vi "fpga.vi"() -> ()   [LabVIEW 2016]
uses:
  <vilib>/rvi/Emulation/niFpgaGetClockAttributes.vi
  <vilib>/rvi/Emulation/niFpgaSctlEmulationGetInTimedLoop.vi
  <vilib>/rvi/Emulation/niFpgaEmulationReportErrorSimple.vi
  <vilib>/rvi/interface/RandomDataEmulation/niFpgaRandomDataHandleErrors.vi
  <vilib>/rvi/Emulation/niFpgaCriticalErrorInLSC.vi
  <vilib>/rvi/eio/common/nirviEmuTemplateMethod_errors.vi
  <vilib>/rvi/DataTransferAndStorage/Container/XNode/niFpgaContainer.xnode
  <vilib>/rvi/interface/RandomDataEmulation/nirviRandomDataFpgaReadWriteTemplate.vi
  <vilib>/eio/EIONode/EIONode.xnode
panel:
  out "bool_arr_out":bool[](array[boolean])
  in  "bool_arr":bool[](array[boolean])=[FALSE, FALSE, FALSE, FALSE, FALSE, FALSE, FALSE, FALSE]
  out "bool_out_7":bool
  out "bool_out_6":bool
  out "bool_out_5":bool
  out "bool_out_4":bool
  out "bool_out_3":bool
  out "bool_out_2":bool
  out "bool_out_1":bool
  out "bool_out_0":bool
  in  "bool_7":bool
  in  "bool_6":bool
  in  "bool_5":bool
  in  "bool_4":bool
  in  "bool_3":bool
  in  "bool_2":bool
  in  "bool_1":bool
  in  "bool_0":bool
  out "indicator_1":sgl
  in  "control_1":sgl
  in  "arr_control":sgl[](array[numeric])=[0.0, 0.0]
  in  "control_0":sgl
  out "arr_indicator":sgl[](array[numeric])
  out "indicator_0":sgl
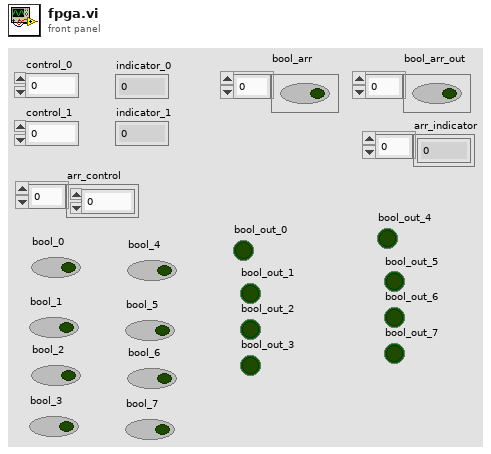
[diagram p1: front panel]
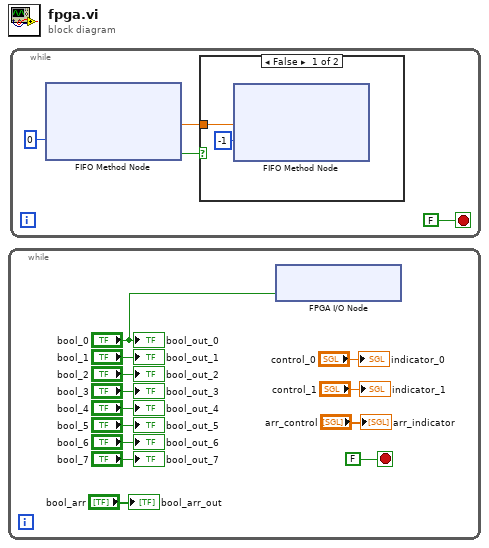
[diagram p0: block diagram]
diagram:
  n1 = while {
    stop <- FALSE stop-if-true
    n2 = xnode "FPGA I/O Node"("USER FPGA LED"="bool_0") -> ()  [unwired: 1 in, 1 out]
    "bool_out_1" <- "bool_1"
    "bool_out_2" <- "bool_2"
    "bool_out_3" <- "bool_3"
    "bool_out_5" <- "bool_5"
    "bool_out_6" <- "bool_6"
    "bool_out_7" <- "bool_7"
    "bool_out_0" <- "bool_0"
    "bool_out_4" <- "bool_4"
    "bool_arr_out" <- "bool_arr"
    "indicator_0" <- "control_0"
    "arr_indicator" <- "arr_control"
    "indicator_1" <- "control_1"
  }
  n3 = while {
    stop <- FALSE stop-if-true
    n4 = xnode ("FIFO Method Node")("Timeout"=0) -> ("Element"=w15:sgl, "Timed Out?"=w16:bool)  [unwired: 1 in, 1 out]
    n5 = case shown="False" w16 {
      tunnel: w15 -> [w18 _]
      frame False {
        n6 = xnode ("FIFO Method Node")("Element"=w18, "Timeout"=-1) -> ()  [unwired: 1 in, 2 out]
      }
      frame True {
      }
    }
  }
